vi "Post-Build Action.vi"(5 "Files Generated by Build":path[](array[path]), 6 "Top Level/Always Included VIs":path[](array[path]), 7 "Destination Path":path, 8 "error in (no error)":errorcluster, 9 "Target Name":string, 10 "Build Specification Name":string, 11 "Project Path":path) -> (0 "error out":errorcluster)   [LabVIEW 2017]
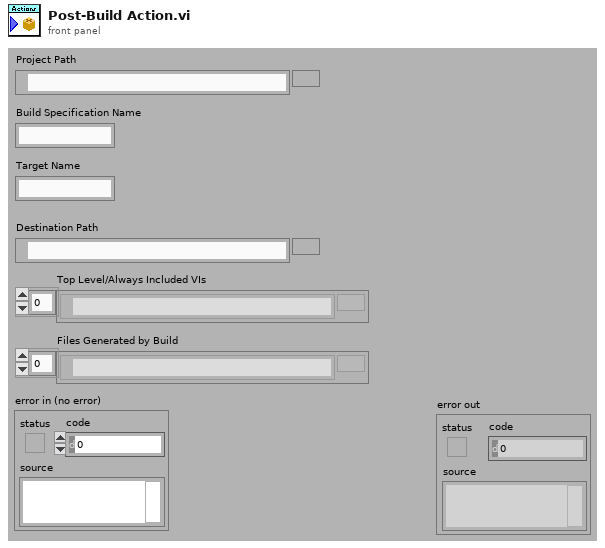
[diagram p1: front panel]
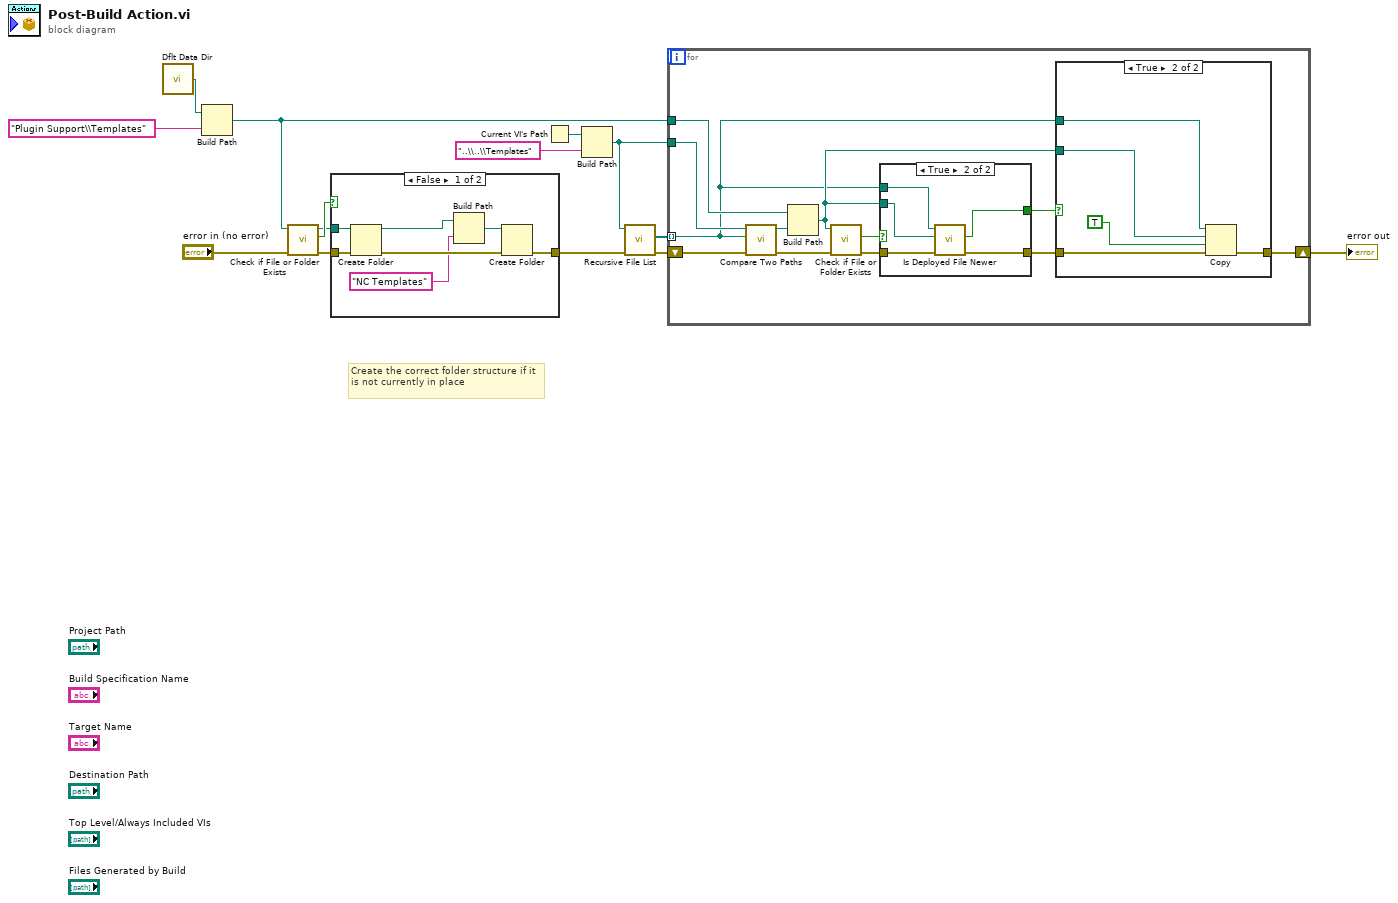
[diagram p0: block diagram]
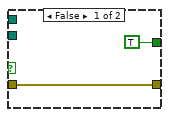
[diagram p3: hidden frame]
diagram:
  # "Create the correct folder structure if it is not currently in place"
  n1 = call <vilib>:"Dflt Data Dir.vi"() -> ("App:Default Data Directory"=w12:path)
  n2 = Build Path(base path=w12, name or relative path="Plugin Support\\Templates") -> (appended path=w6:path)
  n3 = call <vilib>:"Check if File or Folder Exists.vi"("error in (no error)"="error in (no error)", "path"=w6) -> ("error out"=w4:errorcluster, "file or folder exists?"=w5:bool, "dup path"=w2:path)  [unwired: 7 in]
  n4 = case shown="False" w5 {
    tunnel: w4 -> [w21 w22]
    tunnel: [w16 w22] -> w3
    tunnel: w2 -> [w19 _]
    frame False {
      n5 = Create Folder(path (use dialog)=w19, error in=w21) -> (created path=w18:path, error out=w20:errorcluster)  [unwired: 1 in, 1 out]
      n6 = Build Path(base path=w18, name or relative path="NC Templates") -> (appended path=w15:path)
      n7 = Create Folder(path (use dialog)=w15, error in=w20) -> (error out=w16:errorcluster)  [unwired: 1 in, 2 out]
    }
    frame True {
    }
  }
  n8 = Current VI's Path() -> (path=w1:path)
  n9 = Build Path(base path=w1, name or relative path="..\\..\\Templates") -> (appended path=w10:path)
  n10 = call <vilib>:"Recursive File List.vi"("error in (no error)"=w3, "Folder Path"=w10) -> ("error out"=w9:errorcluster, "All Files in Dir"=w11:path[])  [unwired: 5 in, 3 out]
  n11 = for {
    tunnel: w11 -> [w24] mode=indexing
    tunnel: w10 -> [w25]
    tunnel: w6 -> [w26]
    shift-right: [w23] -> w8
    shift-left: w9 -> [w27]
    n12 = call <vilib>:"Compare Two Paths.vi"("error in (no error)"=w27, "Path 2"=w24, "Path 1"=w25) -> ("error out"=w28:errorcluster, "Relative Path from 1 to 2"=w34:path)  [unwired: 5 in, 2 out]
    n13 = Build Path(base path=w26, name or relative path=w34) -> (appended path=w31:path)
    n14 = call <vilib>:"Check if File or Folder Exists.vi"("error in (no error)"=w28, "path"=w31) -> ("error out"=w29:errorcluster, "file or folder exists?"=w33:bool)  [unwired: 7 in, 1 out]
    n15 = case shown="True" w33 {
      tunnel: w24 -> [_ w47]
      tunnel: w31 -> [_ w46]
      tunnel: [TRUE w43] -> w32
      tunnel: [w42 w45] -> w30
      tunnel: w29 -> [w42 w44]
      frame False {
      }
      frame True {
        n16 = call "Is Deployed File Newer.vi"("error in (no error)"=w44, "Deployed Path"=w46, "Template Path"=w47) -> ("error out"=w45:errorcluster, "Deployed Newer?"=w43:bool)  [unwired: 7 in]
      }
    }
    n17 = case shown="True" w32 {
      tunnel: w24 -> [_ w38]
      tunnel: w31 -> [_ w37]
      tunnel: w30 -> [w35 w39]
      tunnel: [w35 w36] -> w23
      frame False {
      }
      frame True {
        n18 = Copy(8:w39, 9:TRUE ("overwrite (F)"), 10:w37, 11:w38) -> (0:w36:errorcluster)  [unwired: 1 in, 2 out]
      }
    }
  }
  "error out" <- w8
